vi "Move To Raw Safe.vi"(8 "error in":errorcluster, 9 "Speed":dbl=5.0, 10 "Destination":refnum<class "Vec3d Class.lvclass">, 11 "Gantry in":refnum<class "Gantry Class.lvclass">) -> (0 "error out":errorcluster, 3 "Gantry out":refnum<class "Gantry Class.lvclass">)   [LabVIEW 2011, in "Gantry Class.lvclass"]
uses:
  Gantry Class.lvclass
  Vec3d Class/Vec3d Class.lvclass
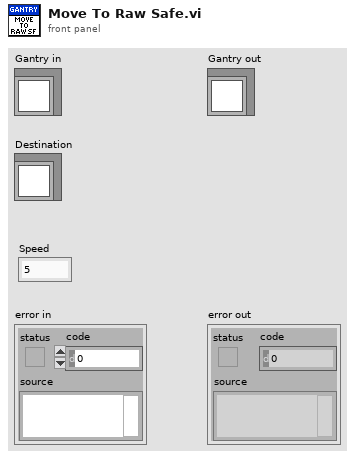
[diagram p1: front panel]
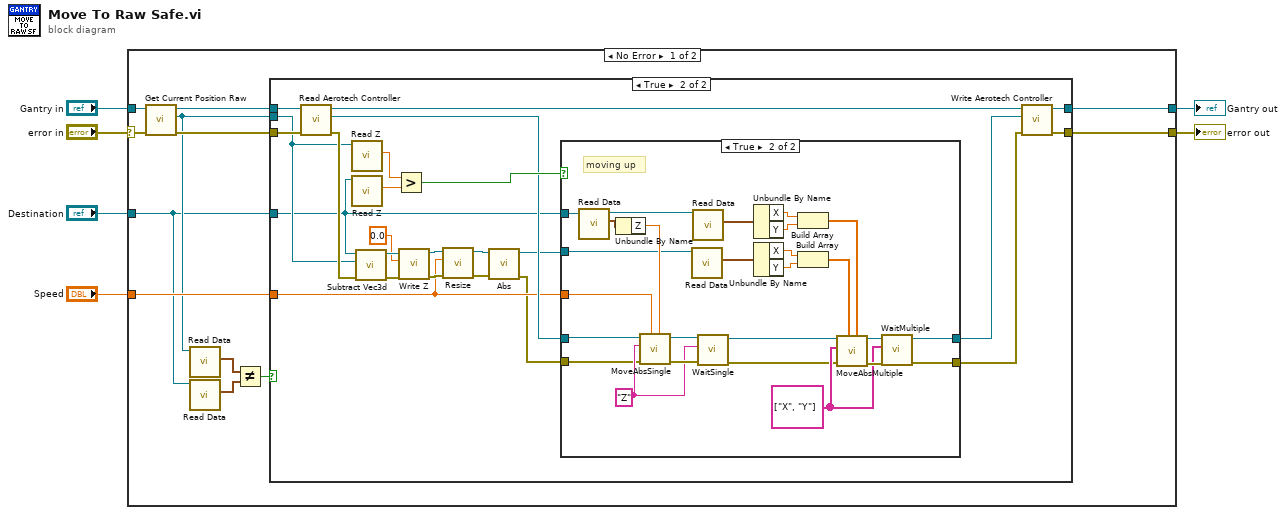
[diagram p0: block diagram]
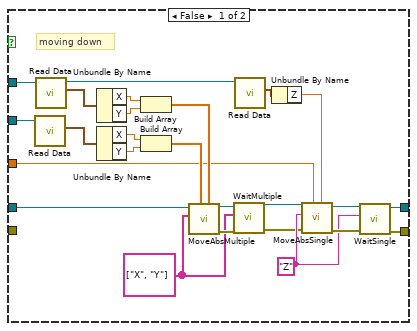
[diagram p3: hidden frame]
diagram:
  n1 = case shown="No Error" "error in" {
    selector: "error in" -> [w13 w97]
    tunnel: [w17 w97] -> w5
    tunnel: [w18 w96] -> w3
    tunnel: "Gantry in" -> [w16 w96]
    tunnel: "Destination" -> [w10 _]
    tunnel: "Speed" -> [w14 _]
    frame No Error {
      n2 = call-dynamic "Get Current Position Raw.vi"("error in (no error)"=w13, "Gantry Class in"=w16) -> ("error out"=w12:errorcluster, "Vec3d Class out"=w11:refnum<class "Vec3d Class.lvclass">, "Gantry Class out"=w15:refnum<class "Gantry Class.lvclass">)  [unwired: 7 in]
      n3 = call-dynamic "Read Data.vi"("Vec3d Class in"=w11) -> ("Data"=w9:cluster{"X":dbl, "Y":dbl, "Z":dbl})  [unwired: 8 in, 2 out]
      n4 = call-dynamic "Read Data.vi"("Vec3d Class in"=w10) -> ("Data"=w8:cluster{"X":dbl, "Y":dbl, "Z":dbl})  [unwired: 8 in, 2 out]
      n5 = Not Equal?(x=w9, y=w8) -> (x != y?=w7:bool)
      n6 = case shown="True" w7 {
        tunnel: [w20 w44] -> w18
        tunnel: [w19 w43] -> w17
        tunnel: w15 -> [w20 w38]
        tunnel: w14 -> [_ w29]
        tunnel: w12 -> [w19 w26]
        tunnel: w11 -> [_ w22]
        tunnel: w10 -> [_ w21]
        frame False {
          # "At destination already, do nothing!"
        }
        frame True {
          n7 = call-dynamic "Read Aerotech Controller.vi"("error in (no error)"=w26, "Gantry Class in"=w38) -> ("error out"=w25:errorcluster, "Aerotech Controller"=w35:refnum<k24>, "Gantry Class out"=w37:refnum<class "Gantry Class.lvclass">)  [unwired: 7 in]
          n8 = call-dynamic "Read Z.vi"("Vec3d Class in"=w22) -> ("Z"=w40:dbl)  [unwired: 8 in, 2 out]
          n9 = call-dynamic "Read Z.vi"("Vec3d Class in"=w21) -> ("Z"=w39:dbl)  [unwired: 8 in, 2 out]
          n10 = call "Subtract Vec3d.vi"("error in (no error)"=w25, "Vec3d in 2"=w22, "Vec3d in 1"=w21) -> ("error out"=w34:errorcluster, "Vec3d Class out"=w33:refnum<class "Vec3d Class.lvclass">)  [unwired: 7 in]
          n11 = Greater?(x=w40, y=w39) -> (0:w36:bool)
          n12 = call-dynamic "Write Z.vi"("error in (no error)"=w34, "Z"=0.0, "Vec3d Class in"=w33) -> ("error out"=w31:errorcluster, "Vec3d Class out"=w30:refnum<class "Vec3d Class.lvclass">)  [unwired: 7 in]
          n13 = call "Resize.vi"("error in"=w31, "length"=w29, "Vec3d in"=w30) -> ("error out"=w24:errorcluster, "Vec3d out"=w28:refnum<class "Vec3d Class.lvclass">)  [unwired: 7 in]
          n14 = call "Abs.vi"("error in"=w24, "Vec3d in"=w28) -> ("error out"=w23:errorcluster, "Vec3d out"=w27:refnum<class "Vec3d Class.lvclass">)  [unwired: 8 in]
          n15 = case shown="True" w36 {
            tunnel: [w60 w94] -> w42
            tunnel: [w59 w92] -> w41
            tunnel: w21 -> [w50 w81]
            tunnel: w35 -> [w63 w85]
            tunnel: w29 -> [w45 w84]
            tunnel: w27 -> [w52 w79]
            tunnel: w23 -> [_ w70]
            frame False {
              w64 = "Z" ("axis name")
              w67 = string[] ["X", "Y"] ("axis names")
              # "moving down"
              n16 = call-dynamic "Read Data.vi"("Vec3d Class in"=w52) -> ("Data"=w57:cluster{"X":dbl, "Y":dbl, "Z":dbl})  [unwired: 8 in, 2 out]
              n17 = call-dynamic "Read Data.vi"("Vec3d Class in"=w50) -> ("Data"=w58:cluster{"X":dbl, "Y":dbl, "Z":dbl}, "Vec3d Class out"=w47:refnum<class "Vec3d Class.lvclass">)  [unwired: 8 in, 1 out]
              n18 = Unbundle By Name(w58) -> ("X"=w56:dbl, "Y"=w55:dbl)
              n19 = Unbundle By Name(w57) -> ("X"=w54:dbl, "Y"=w53:dbl)
              n20 = Build Array(w56, w55) -> (w48:dbl[])
              n21 = Build Array(w54, w53) -> (w49:dbl[])
              n22 = call <userlib>:"MoveAbsMultiple.vi"("positions"=w48, "speeds"=w49, "axis names"=w67, "controller in"=w63) -> ("error out"=w68:errorcluster, "controller out"=w69:refnum<k24>)  [unwired: 6 in]
              n23 = call <userlib>:"WaitMultiple.vi"("error in (no error)"=w68, "axis names"=w67, "controller in"=w69) -> ("error out"=w61:errorcluster, "controller out"=w62:refnum<k24>)  [unwired: 6 in, 1 out]
              n24 = call-dynamic "Read Data.vi"("Vec3d Class in"=w47) -> ("Data"=w51:cluster{"X":dbl, "Y":dbl, "Z":dbl})  [unwired: 8 in, 2 out]
              n25 = Unbundle By Name(w51) -> ("Z"=w46:dbl)
              n26 = call <userlib>:"MoveAbsSingle.vi"("position"=w46, "speed"=w45, "error in (no error)"=w61, "axis name"=w64, "controller in"=w62) -> ("error out"=w65:errorcluster, "controller out"=w66:refnum<k24>)  [unwired: 5 in]
              n27 = call <userlib>:"WaitSingle.vi"("error in (no error)"=w65, "axis name"=w64, "controller in"=w66) -> ("error out"=w59:errorcluster, "controller out"=w60:refnum<k24>)  [unwired: 6 in, 1 out]
            }
            frame True {
              w91 = string[] ["X", "Y"] ("axis names")
              w86 = "Z" ("axis name")
              # "moving up"
              n28 = call-dynamic "Read Data.vi"("Vec3d Class in"=w81) -> ("Data"=w83:cluster{"X":dbl, "Y":dbl, "Z":dbl}, "Vec3d Class out"=w80:refnum<class "Vec3d Class.lvclass">)  [unwired: 8 in, 1 out]
              n29 = Unbundle By Name(w83) -> ("Z"=w82:dbl)
              n30 = call <userlib>:"MoveAbsSingle.vi"("position"=w82, "speed"=w84, "error in (no error)"=w70, "axis name"=w86, "controller in"=w85) -> ("error out"=w88:errorcluster, "controller out"=w90:refnum<k24>)  [unwired: 5 in]
              n31 = call-dynamic "Read Data.vi"("Vec3d Class in"=w79) -> ("Data"=w77:cluster{"X":dbl, "Y":dbl, "Z":dbl})  [unwired: 8 in, 2 out]
              n32 = call-dynamic "Read Data.vi"("Vec3d Class in"=w80) -> ("Data"=w78:cluster{"X":dbl, "Y":dbl, "Z":dbl})  [unwired: 8 in, 2 out]
              n33 = call <userlib>:"WaitSingle.vi"("error in (no error)"=w88, "axis name"=w86, "controller in"=w90) -> ("error out"=w87:errorcluster, "controller out"=w89:refnum<k24>)  [unwired: 6 in, 1 out]
              n34 = Unbundle By Name(w78) -> ("X"=w76:dbl, "Y"=w75:dbl)
              n35 = Unbundle By Name(w77) -> ("X"=w74:dbl, "Y"=w73:dbl)
              n36 = Build Array(w76, w75) -> (w71:dbl[])
              n37 = Build Array(w74, w73) -> (w72:dbl[])
              n38 = call <userlib>:"MoveAbsMultiple.vi"("positions"=w71, "speeds"=w72, "error in (no error)"=w87, "axis names"=w91, "controller in"=w89) -> ("error out"=w93:errorcluster, "controller out"=w95:refnum<k24>)  [unwired: 5 in]
              n39 = call <userlib>:"WaitMultiple.vi"("error in (no error)"=w93, "axis names"=w91, "controller in"=w95) -> ("error out"=w92:errorcluster, "controller out"=w94:refnum<k24>)  [unwired: 6 in, 1 out]
            }
          }
          n40 = call-dynamic "Write Aerotech Controller.vi"("error in (no error)"=w41, "Aerotech Controller"=w42, "Gantry Class in"=w37) -> ("error out"=w43:errorcluster, "Gantry Class out"=w44:refnum<class "Gantry Class.lvclass">)  [unwired: 7 in]
        }
      }
    }
    frame Error {
    }
  }
  "error out" <- w5
  "Gantry out" <- w3
